vi "相机1-保存当前图片为放螺丝时PCB孔槽参考图片.vi"(9 "拍PCB孔功能":enum16{"存储校准时影像", "计算放螺丝时补偿量"}(ring), 11 "Image In":T3) -> (0 "机械手移动量 mm":T1 {"X" format="%#.3f"}, 2 "相机1校准时拍PCB影像坐标":T1 {"X" format="%#.3f"}, 3 "Image":T3(plugin-control))   [LabVIEW 2014]
uses:
  Global.vi
  <vilib>/vision/Measure.llb/Edge Polarity.ctl
  <vilib>/vision/Measure.llb/Edge Options.ctl
  <vilib>/vision/Image Controls.llb/IMAQ Image.ctl
  Controls/XYPos.ctl
panel:
  out "图像偏差量 Pixles":T1 {"X" format="%#.3f"}
  in  "显示内容":string[](array[string])=["机械手补偿量-X", "机械手补偿量-Y", "机械手补偿量-角度"]
  in  "量测项目名称":string[](array[string])=["校准时影像坐标-X", "校准时影像坐标-Y", "校准时影像坐标-角度"]
  in  "Img Path":path=path "C:/Users/aicter/Desktop/上相机对位时Gold影像.png"
  out "Fitted Circle":T2 {"Average SNR (dB)" format="%.2f"; "Average Strength" format="%.2f"; "Roundness (Real-World)" format="%.2f"; "Radius (Real-World)" format="%.2f"; "Center (Real-World)"."Y" format="%.2f"; "Center (Real-World)"."X" format="%.2f"; "Radius (Pixels)" format="%.2f"; "Center (Pixels)"."Y" format="%.2f"; "Center (Pixels)"."X" format="%.2f"}
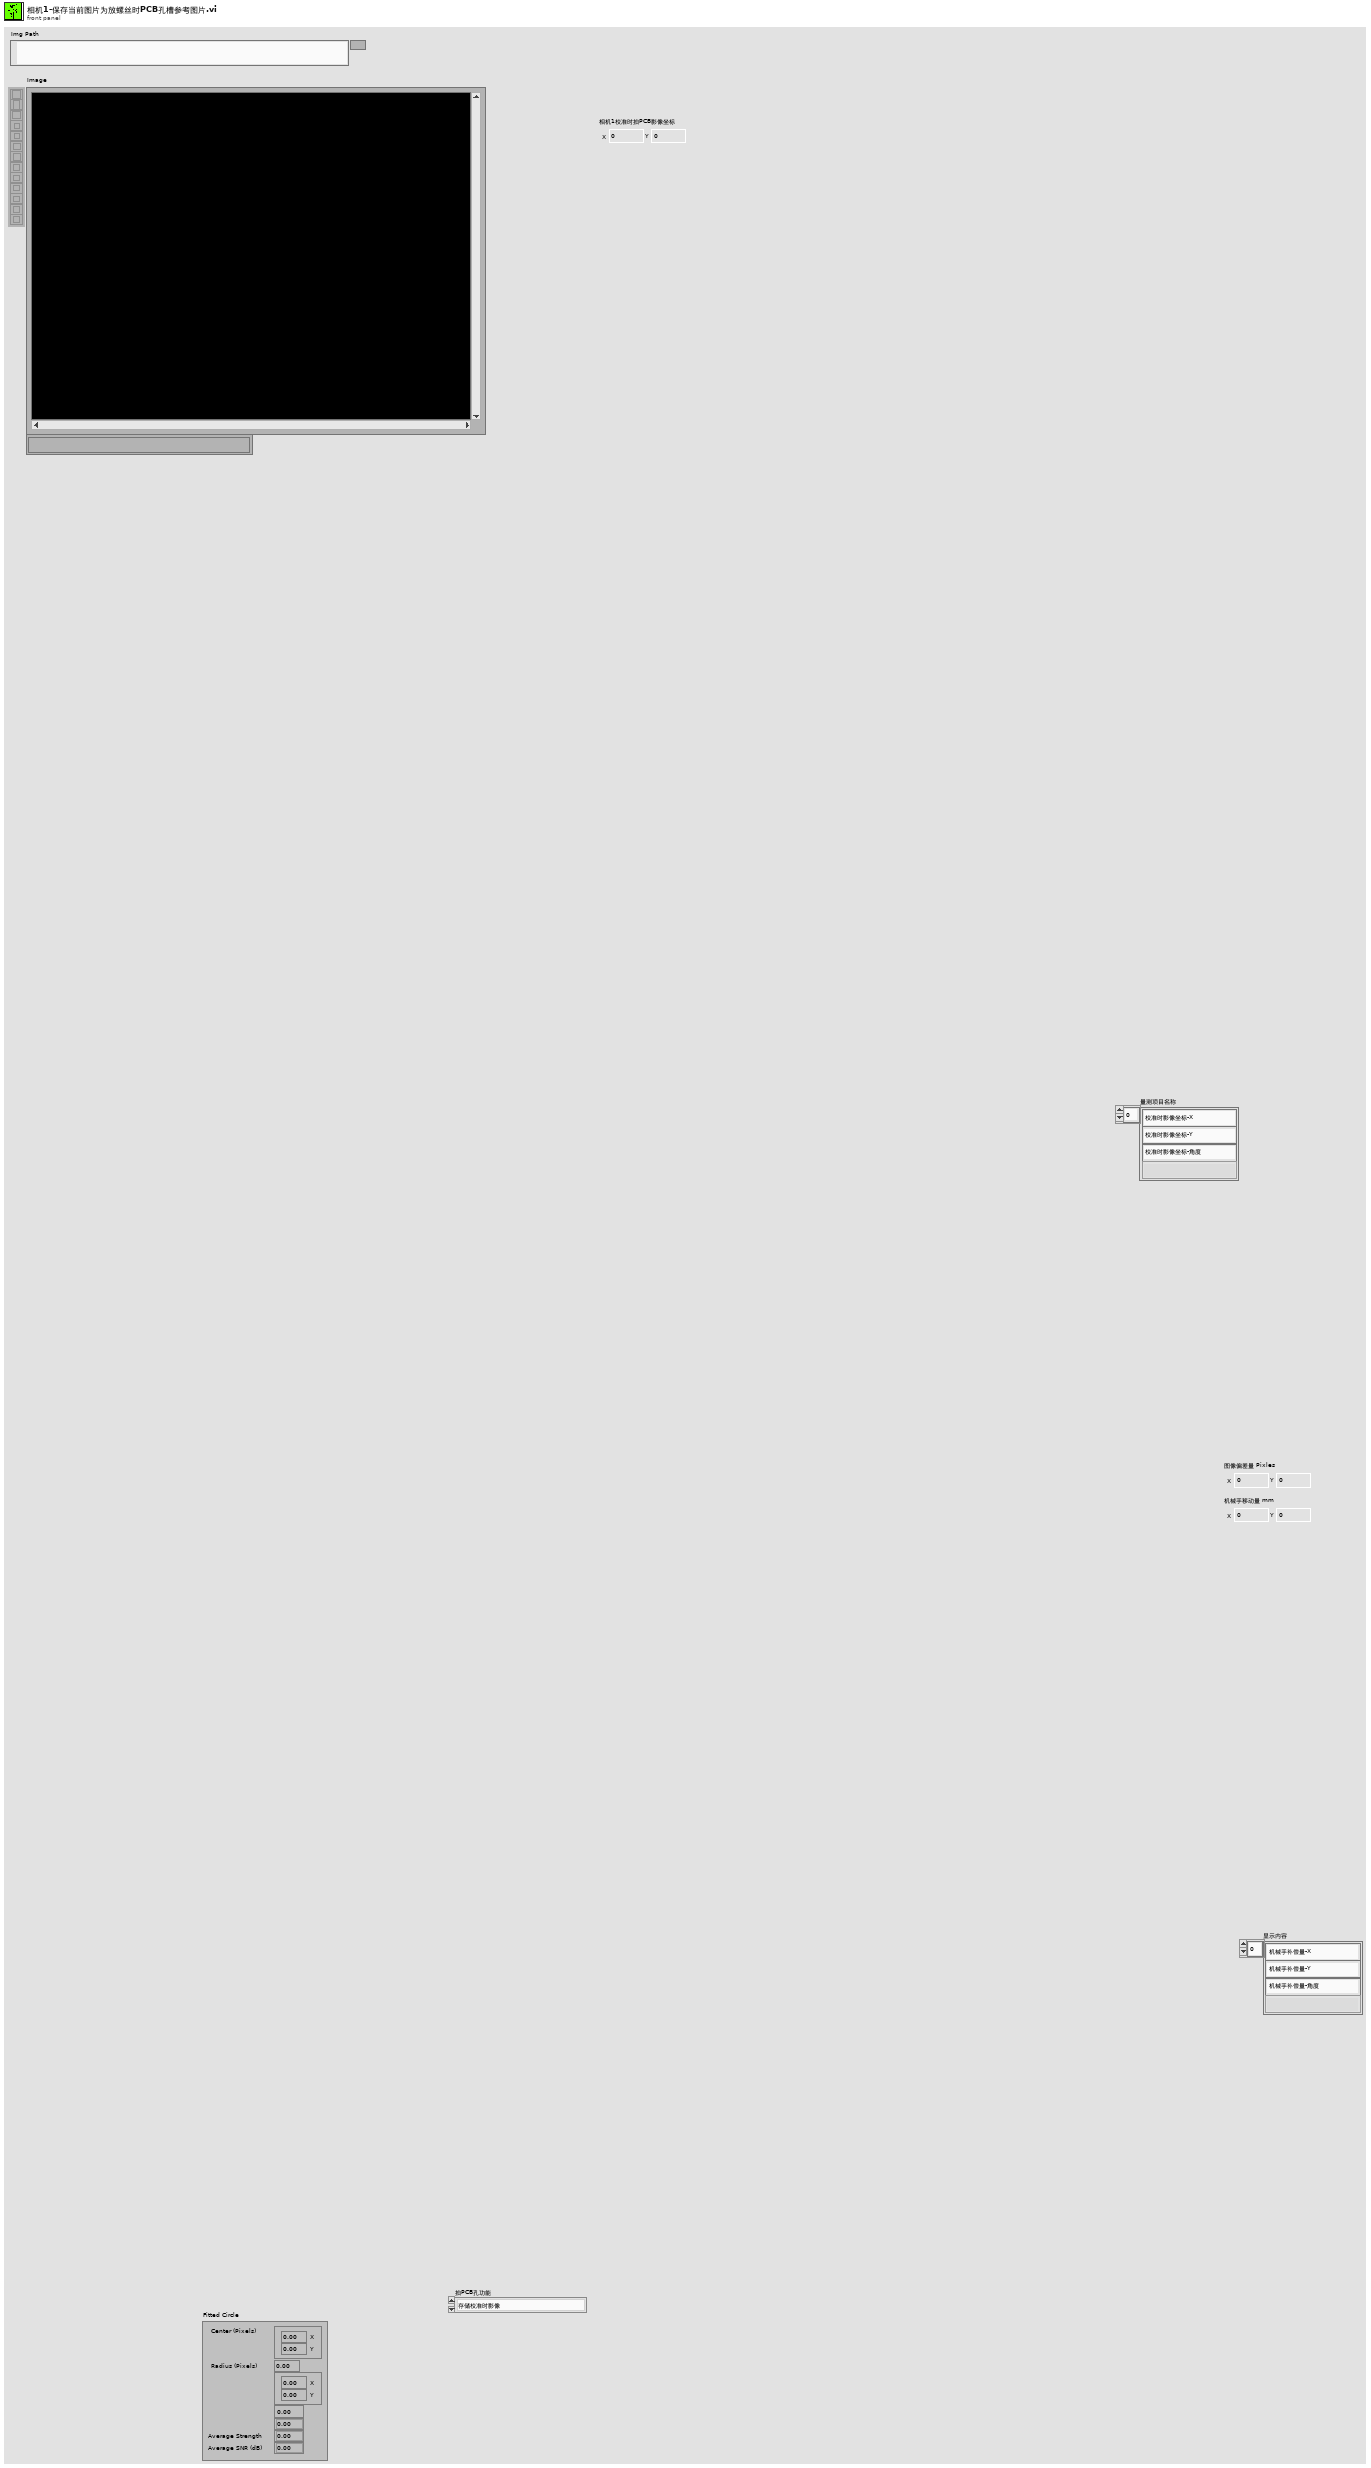
[diagram p1: front panel]
types:
  T1 = typedef "XYPos.ctl" = cluster{"X":dbl, "Y":dbl}
  T2 = cluster{"Center (Pixels)":cluster{"X":sgl, "Y":sgl}, "Radius (Pixels)":dbl, "Center (Real-World)":cluster{"X":sgl, "Y":sgl}, "Radius (Real-World)":dbl, "Roundness (Real-World)":dbl, "Average Strength":dbl, "Average SNR (dB)":dbl}
  T3 = typedef "IMAQ Image.ctl" = refnum<image>
  T4 = typedef "Edge Options.ctl" = cluster{"Edge Polarity":T5, "Kernel Size":u32, "Width":u32, "Minimum Edge Strength":sgl, "Interpolation Type":enum32{"Zero Order", "Bilinear", "Quadratic", "Cubic", "Bilinear Fixed"}, "Data Processing Method":enum32{"Average", "Median"}}
  T5 = typedef "Edge Polarity.ctl" = u32
  T6 = cluster{"Search  Direction":u32, "Edge Options":T4, "Show Search Area":bool, "Show Search Lines":bool, "Show Edges Found":bool, "Show Result":bool, "Search Area Color":u32, "Search Lines Color":u32, "Edge Locations Color":u32, "Result Color":u32, "Overlay Group Name":string}
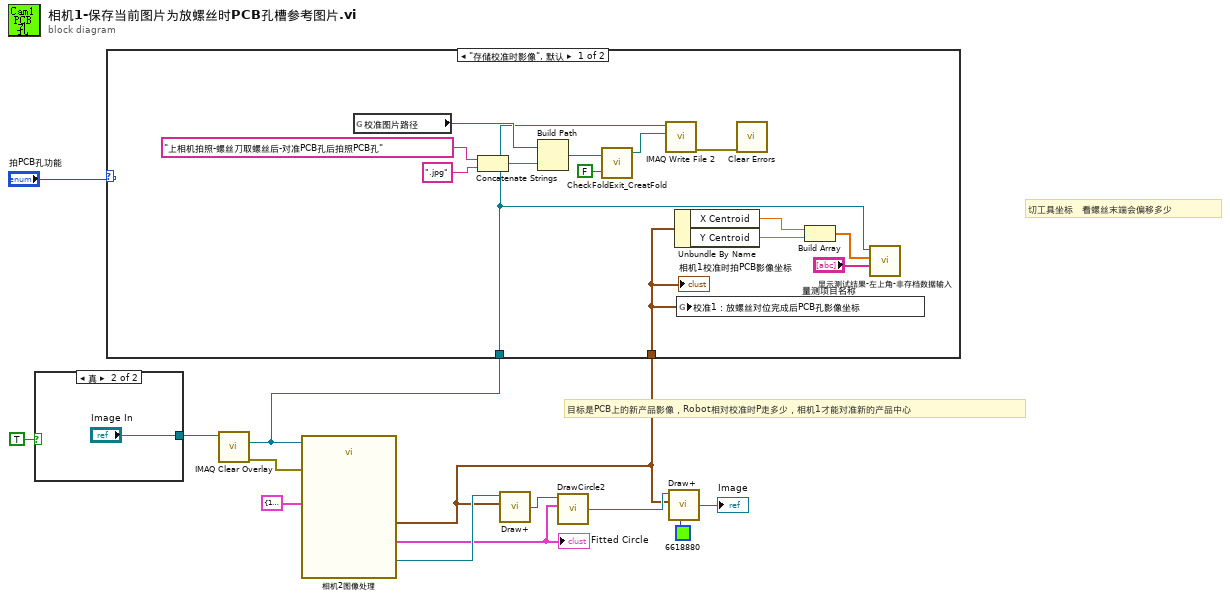
[diagram p0: block diagram]
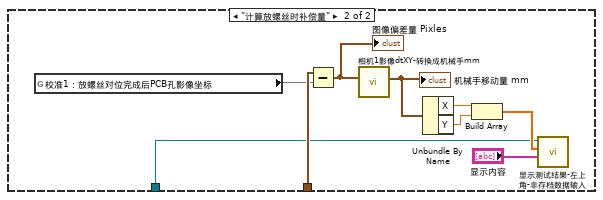
[diagram p2: hidden frame]
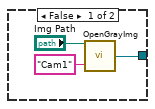
[diagram p3: hidden frame]
diagram:
  # "切工具坐标   看螺丝末端会偏移多少"
  # "目标是PCB上的新产品影像，Robot相对校准时P走多少，相机1才能对准新的产品中心"
  n1 = case shown="真" TRUE {
    tunnel: [w16 "Image In"] -> w7
    frame False {
      n2 = call "OpenGrayImg.vi"("Image Name"="Cam1", "Img Path"="Img Path") -> ("Image Out"=w16:T3)
    }
    frame True {
    }
  }
  n3 = call "IMAQ Clear Overlay"("Image"=w7) -> ("error out"=w6:errorcluster, "Image Out"=w4:T3)  [unwired: 9 in]
  n4 = call "相机2图像处理"("Image In"=w4, "Options (Find Circular Edge 1)"=T6 {"Search  Direction"=1, "Edge Options"={"Edge Polarity"=0, "Kernel Size"=7, "Width"=3, "Minimum Edge Strength"=30.0, "Interpolation Type"=enum."Bilinear Fixed", "Data Processing Method"=enum."Average"}, "Show Search Area"=FALSE, "Show Search Lines"=FALSE, "Show Edges Found"=FALSE, "Show Result"=TRUE, "Search Area Color"=65280, "Search Lines Color"=255, "Edge Locations Color"=16776960, "Result Color"=16711680, "Overlay Group Name"=""}, "error in"=w6) -> ("Image Out"=w12:T3, "Centroid (Centroid 1)"=w1:cluster{"X Centroid":sgl, "Y Centroid":sgl}, "Fitted Circle (Find Circular Edge 1)"=w8:T2)  [unwired: 21 in, 1 out]
  "Fitted Circle" <- w8
  n5 = case shown="\"存储校准时影像\", 默认" "拍PCB孔功能" {
    tunnel: w4 -> [w19 w32]
    tunnel: w1 -> [w18 w38]
    frame "存储校准时影像", Default {
      n6 = global read "Global.vi" "校准图片路径"() -> (w31:path)
      n7 = Concatenate Strings("上相机拍照-螺丝刀取螺丝后-对准PCB孔后拍照PCB孔" ("time format string (%c)"), ".jpg" ("字符串")) -> (w30:string)
      n8 = Build Path(base path=w31, name or relative path=w30) -> (appended path=w26:path)
      n9 = call "CheckFoldExit_CreatFold.vi"("path in"=w26, "FoldOrFile¡H"=FALSE) -> ("File out"=w24:path)  [unwired: 2 out]
      n10 = call-poly "IMAQ Write File 2"("File Path"=w24, "Image"=w19) -> ("error out"=w29:errorcluster)  [unwired: 8 in, 1 out]
      n11 = Unbundle By Name(w18) -> ("X Centroid"=w22:sgl, "Y Centroid"=w23:sgl)
      n12 = global write "Global.vi" "校准1：放螺丝对位完成后PCB孔影像坐标"(w18) -> ()
      n13 = call <vilib>:"Clear Errors.vi"("error in (no error)"=w29) -> ()  [unwired: 5 in, 2 out]
      n14 = Build Array(w22, w23) -> (w21:sgl[])
      n15 = call "显示测试结果-左上角-非存档数据输入.vi"("量测项目名称"="量测项目名称", "显示数据"=w21, "Img输入"=w19) -> ()  [unwired: 8 in, 1 out]
      "相机1校准时拍PCB影像坐标" <- w18
    }
    frame "计算放螺丝时补偿量" {
      n16 = global read "Global.vi" "校准1：放螺丝对位完成后PCB孔影像坐标"() -> (w37)
      n17 = Subtract(x=w38, y=w37) -> (x-y=w39:cluster{"X Centroid":sgl, "Y Centroid":sgl})
      "图像偏差量 Pixles" <- w39
      n18 = call "相机1影像dtXY-转换成机械手mm.vi"("校准：相机1示教时影像坐标"=w39) -> ("机械手移动量 mm"=w40:T1)  [unwired: 9 in, 1 out]
      "机械手移动量 mm" <- w40
      n19 = Unbundle By Name(w40) -> ("X"=w35:dbl, "Y"=w34:dbl)
      n20 = Build Array(w35, w34) -> (w33:dbl[])
      n21 = call "显示测试结果-左上角-非存档数据输入.vi"("量测项目名称"="显示内容", "显示数据"=w33, "Img输入"=w32) -> ()  [unwired: 8 in, 1 out]
    }
  }
  n22 = call "Draw+.vi"("input cluster"=w1, "Image In"=w12) -> ("Image Out"=w10:T3)  [unwired: 4 in]
  n23 = call "DrawCircle2.vi"("Fitted Circle (左圆)"=w8, "Img in"=w10) -> ("Img out"=w11:T3)  [unwired: 2 in]
  n24 = call "Draw+.vi"("Color"=u32 6618880, "input cluster"=w1, "Image In"=w11) -> ("Image Out"=→"Image":T3)  [unwired: 3 in]
